vi "EndSubRoutine.vi"(0 "Done?":bool, 2 "Ran too long?":bool) -> (6 "Safe Stop?":bool, 7 "Stop?":bool)   [LabVIEW 2017]
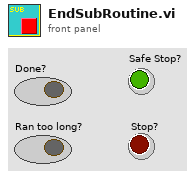
[diagram p1: front panel]
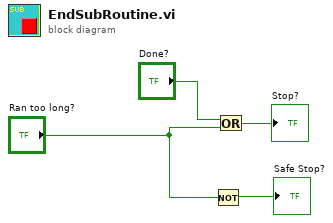
[diagram p0: block diagram]
diagram:
  n1 = Not(x="Ran too long?") -> (.not. x?=→"Safe Stop?":bool)
  n2 = Or(x="Done?", y="Ran too long?") -> (x .or. y?=→"Stop?":bool)
